vi "Serial Terminal Write.vi"() -> ()   [LabVIEW 2025]
doc: "This example shows how to do basic serial write communication.\n\nThis example expects a serial cable connected from your development PC to the RS-232 connector on the roboRIO.\n\nNote: before using this example with RS-232 you must turn off Console Out on the roboRIO. This can be done in the roboRIO Imaging Tool."
uses:
  <vilib>/Rock Robotics/WPI/SerialPort/WPI_SerialPort.ctl
panel:
  in  "Serial Port":T1
  in  "write":bool
  in  "stop":bool
  out "error out":errorcluster
  out "Bytes Written":u32
  in  "Text to Write":string="Testing FRC serial write message. Can you read it?"
  in  "Flow Control":u16(ring) items=["None", "XON/XOFF", "RTS/CTS", "XON/XOFF & RTS/CTS", "DTR/DSR", "XON/XOFF & DTR/DSR"]
  in  "Stop Bits":u16(ring)=10 items=["1.0"=10, "1.5"=15, "2.0"=20]
  in  "Parity":u16(ring) items=["None", "Odd", "Even", "Mark", "Space"]
  in  "Data Bits":u16=8
  in  "Baud Rate":u32=115200
  # "Set these inputs before running."
  # "Controls and Output"
  # "Note: before using this example you must turn off Console Out on the roboRIO.  This can be done in the roboRIO Imaging Tool"
  # "This shows wiring for serial communication.  Plug the female DB-9 connector into your PC, and then use a serial console such as PuTTY for communication testing."
  # "Female DB-9 Pinout\nfront view"
  # "DB-9\n2 (white wire)------\n3 (red wire)--------\n5 (black wire)------"
  # "roboRIO\nRS-232 TXD\nRS-232 RXD\nRS-232"
  # "5"
  # "4"
  # "3"
  # "2"
  # "1"
  # "9"
  # "8"
  # "7"
  # "6"
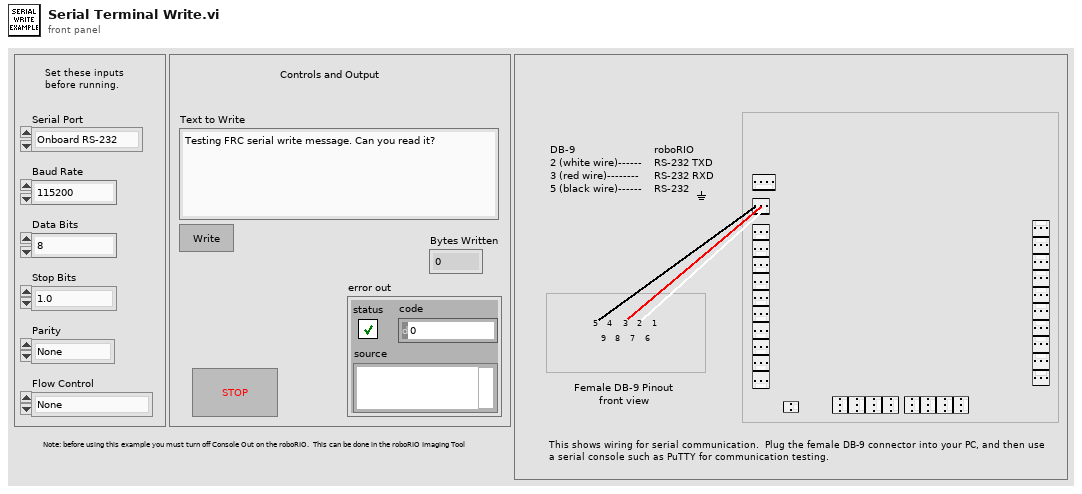
[diagram p1: front panel]
types:
  T1 = typedef "WPI_SerialPort.ctl" = enum16{"Onboard RS-232", "MXP TTL", "USB 1", "USB 2"}
  T2 = typedef "WPI_SerialPortRef.ctl" = cluster{"DevStatus":errorcluster, "Serial Port Name":refnum<visa-resource-name>}
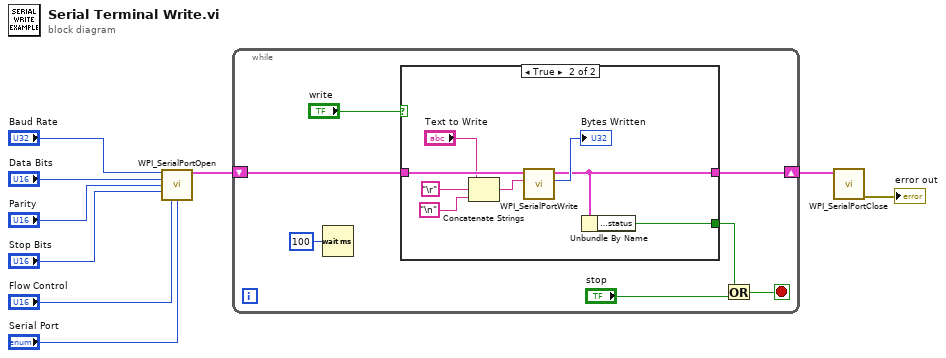
[diagram p0: block diagram]
diagram:
  n1 = call <vilib>:"WPI_SerialPortOpen.vi"("Baud Rate"="Baud Rate", "Data Bits"="Data Bits", "Parity"="Parity", "Stop Bits"="Stop Bits", "Flow Control"="Flow Control", "Serial Port"="Serial Port") -> ("SerialPortRef"=w4:T2)  [unwired: 8 in, 1 out]
  n2 = while {
    shift-right: [w14] -> w3
    shift-left: w4 -> [w16]
    stop <- w13 stop-if-true
    n3 = Wait (ms)(milliseconds to wait=u32 100) -> ()  [unwired: 1 out]
    n4 = case shown="True" "write" {
      tunnel: w16 -> [w17 w25]
      tunnel: [w17 w20] -> w14
      tunnel: [_ w19] -> w10
      frame False {
      }
      frame True {
        n5 = Concatenate Strings("Text to Write", "\r", "\n") -> (w21:string)
        n6 = call <vilib>:"WPI_SerialPortWrite.vi"("Buffer"=w21, "SerialPortRef"=w25) -> ("Num Bytes Written"=→"Bytes Written":u32, "SerialPortRef"=w20:T2)  [unwired: 7 in, 1 out]
        n7 = Unbundle By Name(w20) -> ("DevStatus.status"=w19:bool)
      }
    }
    n8 = Or(x=w10, y="stop") -> (x .or. y?=w13:bool)
  }
  n9 = call <vilib>:"WPI_SerialPortClose.vi"("SerialPortRef"=w3) -> ("error out"=→"error out":errorcluster)  [unwired: 10 in]
